vi "Set Pressure Sensor Settings.vi"(10 "Pressure Sensor Settings":T1 {"Offset" format="%_6f"; "PSI per Volt" format="%_6f"}, 11 "Model in":refnum<class "Model.lvclass">) -> (3 "Model out":refnum<class "Model.lvclass">)   [LabVIEW 2015, in "Model.lvclass"]
uses:
  Model.lvclass
  Typedefs/Pressure Sensor Settings.ctl
  Model.lvclass/Model.ctl
  Typedefs/FAMT Typedefs.lvlib
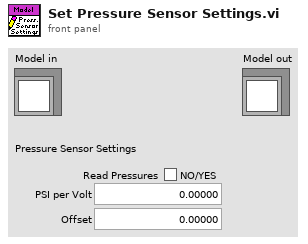
[diagram p1: front panel]
types:
  T1 = typedef "FAMT Typedefs.lvlib/Pressure Sensor Settings.ctl" = cluster{"Read Pressures":bool, "PSI per Volt":dbl, "Offset":dbl}
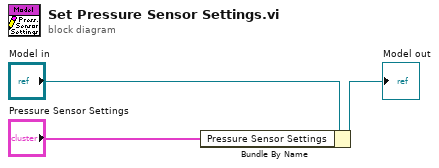
[diagram p0: block diagram]
diagram:
  n1 = Bundle By Name(cluster="Model in", "Pressure Sensor Settings"="Pressure Sensor Settings") -> (→"Model out":refnum<class "Model.lvclass">)
